vi "CT400_testwrap.vi"() -> ()   [LabVIEW 2013]
uses:
  CT400_Lib/CT400_lib.lvlib
panel:
  out "Error Init":i32
  in  "Laser Type":u32(ring) items=["LS_TunicsPlus", "LS_TunicsPurity", "LS_TunicsReference", "LS_TunicsT100s_HP", "LS_TunicsT100r", "LS_JdsuSws", "LS_Agilent", "NB_SOURCE"]
  out "CT400 Option":string
  out "# Spectral Lines":i32
  out "Spectral lines":dbl[](array[numeric]) format="%#.4f"
  in  "Resolution [pm]":u32=2 max=128 step=1
  out "#Nb of available \ndetectors":i32
  out "# Nb of available\ninputs":i32
  out "# of acquired points":i32
  out "Vext out":dbl format="%.4g"
  out "# of resampled points":i32
  out "Pout-interpolated":dbl[](array[numeric]) format="%.2g"
  out "Detector-interpolated":dbl[](array[numeric]) format="%.2g"
  out "Wavelength re-sampled":dbl[](array[numeric]) format="%.3g"
  in  "Interpolated data":string="Detector1_output-resampled.txt"
  in  "Re-sampled wavelength":string="Wavelength-resampled.txt"
  in  "Detector data":string="Detector1_output.txt"
  in  "Wavelength data":string="Wavelength.txt"
  out "Pout":dbl[](array[numeric]) format="%.2g"
  out "Detector":dbl[](array[numeric]) format="%#.2g"
  out "Wavelength":dbl[](array[numeric]) format="%.4f"
  out "P4 [dBm]":dbl format="%.2g"
  out "P3 [dBm]":dbl format="%.2g"
  out "P2 [dBm]":dbl format="%.2g"
  out "P1 [dBm]":dbl format="%.2g"
  out "Pout [dBm]":dbl format="%.2g"
  out "Error/warning":string
  out "error out":errorcluster
  in  "Start Wavelength [nm]":dbl=1490.0
  in  "Laser power output [mW]":dbl=1.0
  in  "Stop Wavelength [nm]":dbl=1640.0
  in  "Speed [nm/s]":i32=50
  in  "GPIB Address":i32=10
  in  "Upper Wavelength [nm]":dbl=1640.0
  in  "Lower Wavelength [nm]":dbl=1490.0
  in  "error in (no error)":errorcluster
  # "CT400 Settings"
  # "Data files (relative path)"
  # "Laser Settings"
  # "Power on detectors"
  # "Re-sampled Measurements"
  # "Measurements"
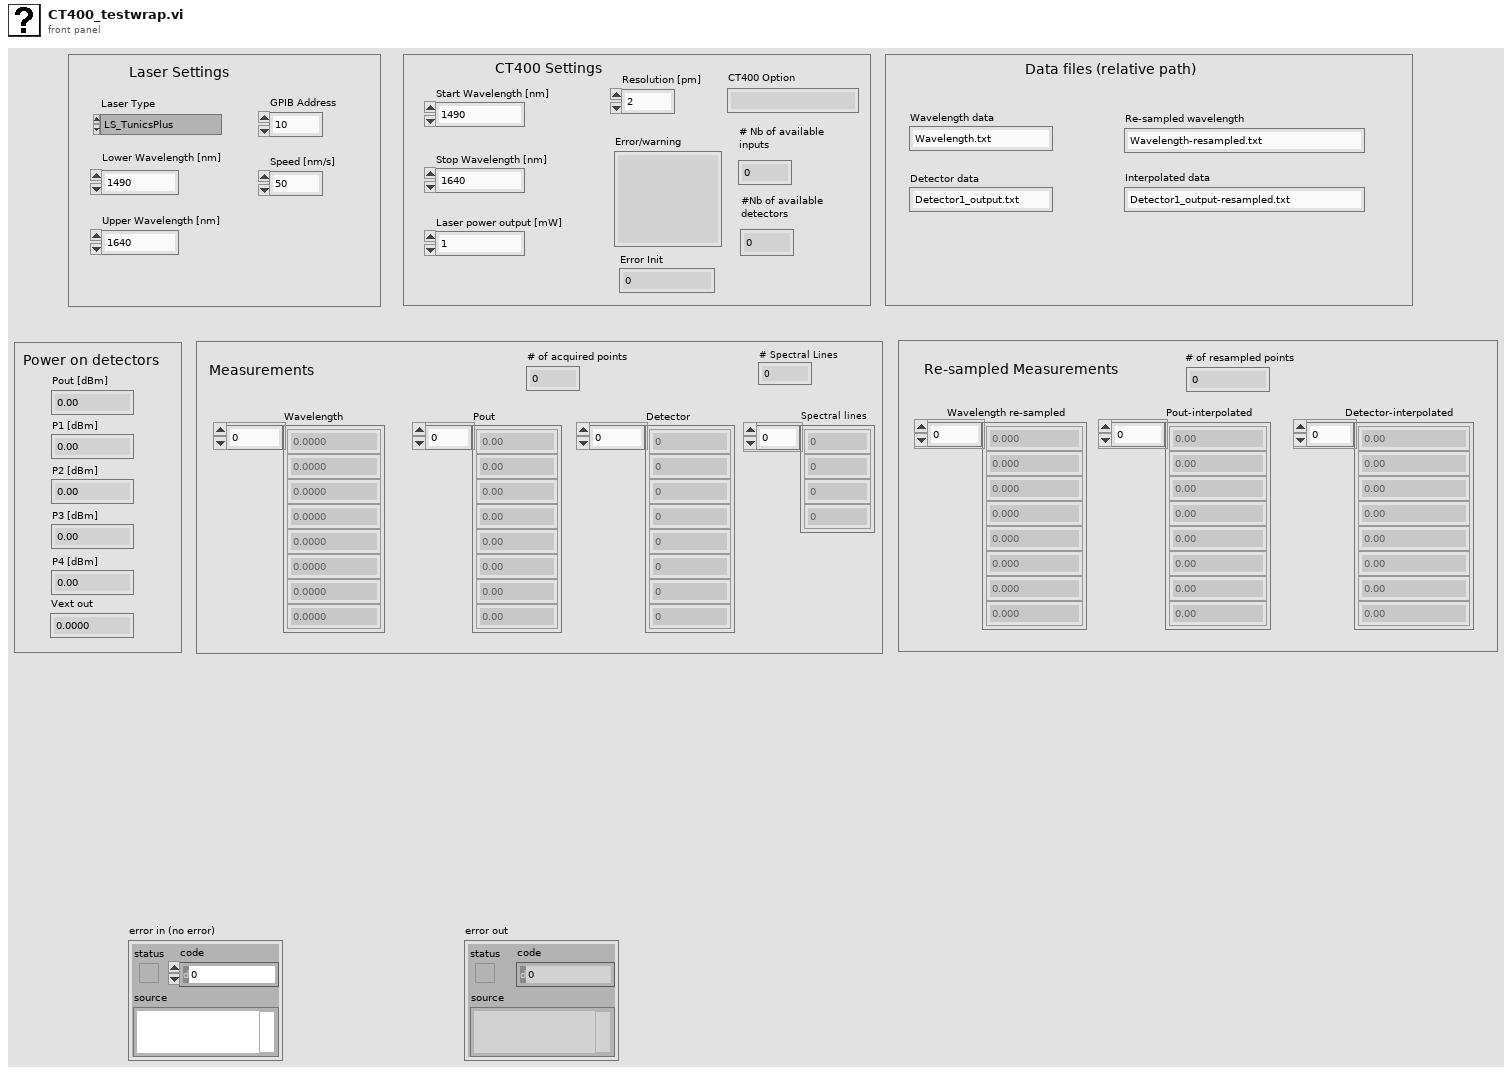
[diagram p1: front panel]
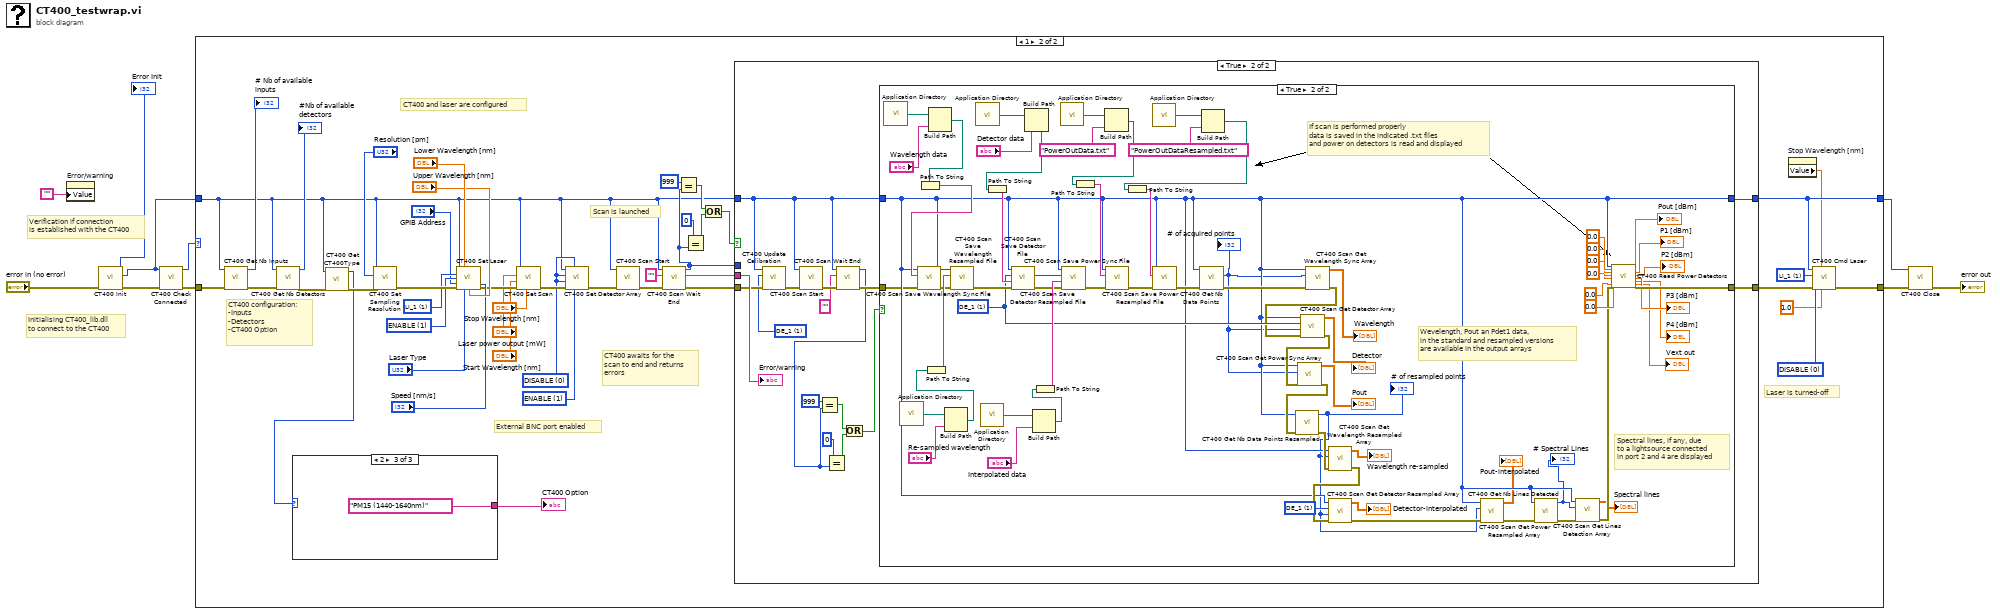
[diagram p0: block diagram]
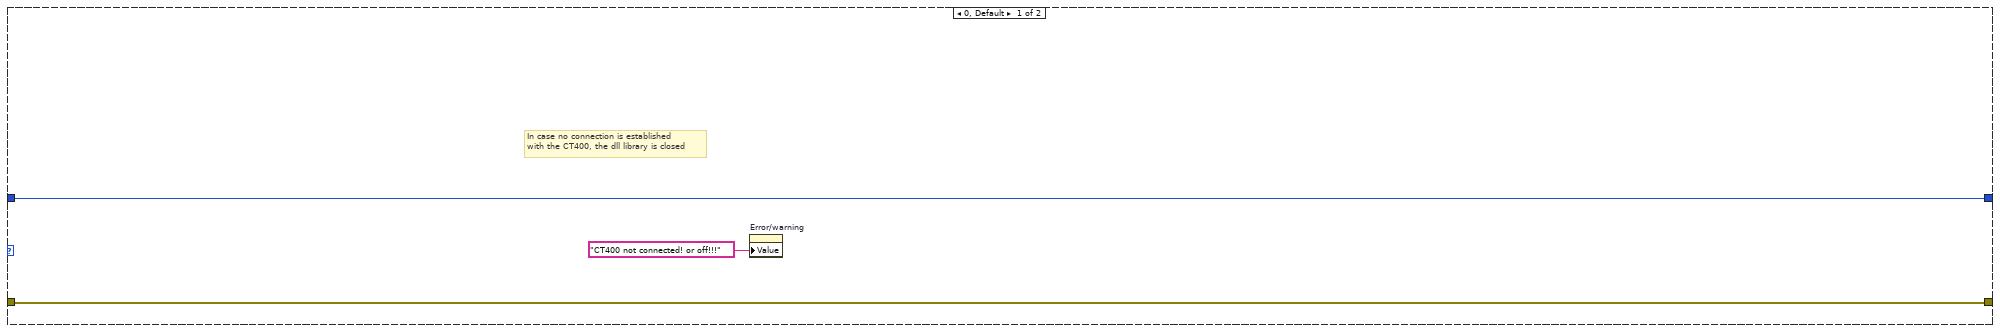
[diagram p2: hidden frame]
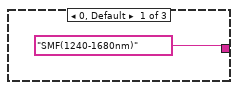
[diagram p3: hidden frame]
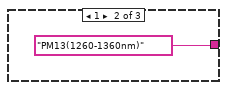
[diagram p4: hidden frame]
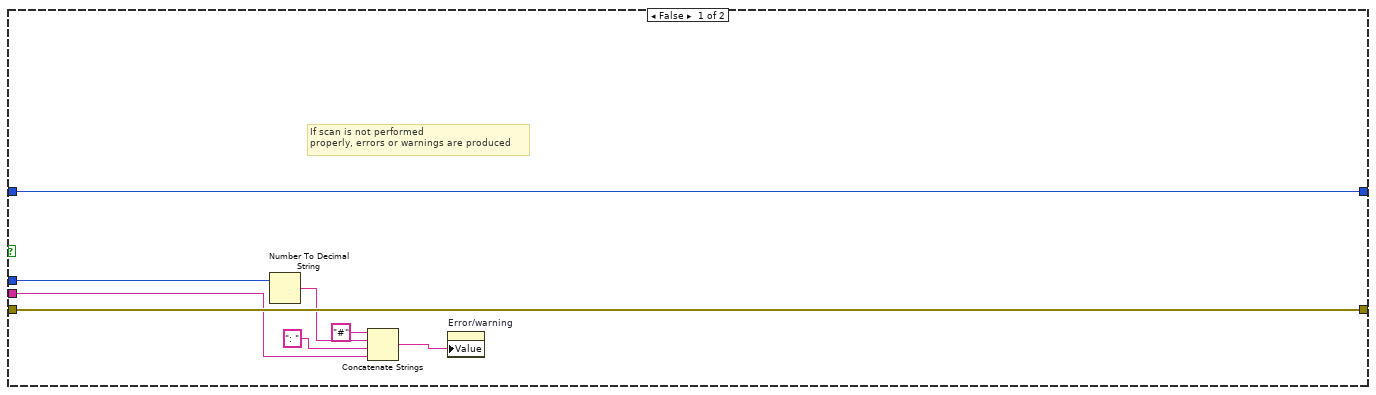
[diagram p5: hidden frame]
diagram:
  # "Verification if connection\nis established with the CT400"
  # "Initialising CT400_lib.dll\nto connect to the CT400"
  n1 = property on="Error/warning" class="Str"("Value"="") -> ()  [unwired: 2 in, 2 out]
  n2 = call "CT400 Init.vi"("error in (no error)"="error in (no error)") -> ("error out"=w9:errorcluster, "function return"=w2:u64, "iError out"=→"Error Init":i32)  [unwired: 8 in]
  n3 = call "CT400 Check Connected.vi"("error in (no error)"=w9, "uiHandle"=w2) -> ("error out"=w7:errorcluster, "function return"=w8:i32)  [unwired: 8 in]
  n4 = case shown="1" w8 {
    tunnel: [w13 w41] -> w6
    tunnel: w7 -> [w13 w25]
    tunnel: [w12 w40] -> w5
    tunnel: w2 -> [w12 w18]
    frame 0, Default {
      # "In case no connection is established\nwith the CT400, the dll library is closed"
      n5 = property on="Error/warning" class="Str"("Value"="CT400 not connected! or off!!!" ("Error/warning")) -> ()  [unwired: 2 in, 2 out]
    }
    frame 1 {
      w14 = u32 1 items=["DISABLE", "ENABLE"] ("eExt")
      w26 = u32 0 items=["DISABLE", "ENABLE"] ("eDect4")
      w38 = u32 1 items=["LI_1"=1, "LI_2"=2, "LI_3"=3, "LI_4"=4] ("eLaser")
      w39 = u32 0 items=["DISABLE", "ENABLE"] ("eEnable")
      w54 = u32 1 items=["DISABLE", "ENABLE"] ("eEnable")
      w55 = u32 1 items=["LI_1"=1, "LI_2"=2, "LI_3"=3, "LI_4"=4] ("eLaser")
      # "CT400 configuration:\n-Inputs\n-Detectors\n-CT400 Option"
      # "External BNC port enabled"
      # "Laser is turned-off"
      # "CT400 awaits for the\nscan to end and returns\nerrors"
      # "Scan is launched"
      # "CT400 and laser are configured"
      n6 = call "CT400 Get Nb Inputs.vi"("error in (no error)"=w25, "uiHandle"=w18) -> ("error out"=w23:errorcluster, "function return"=→"# Nb of available\ninputs":i32)  [unwired: 8 in]
      n7 = call "CT400 Get Nb Detectors.vi"("error in (no error)"=w23, "uiHandle"=w18) -> ("error out"=w19:errorcluster, "function return"=→"#Nb of available \ndetectors":i32)  [unwired: 8 in]
      n8 = call "CT400 Get CT400Type.vi"("error in (no error)"=w19, "uiHandle"=w18) -> ("error out"=w20:errorcluster, "function return"=w17:i32)  [unwired: 8 in]
      n9 = case shown="2" w17 {
        tunnel: ["SMF(1240-1680nm)" ("CT400 Option") "PM13(1260-1360nm)" ("CT400 Option") "PM15 (1440-1640nm)" ("CT400 Option")] -> w16
        frame 0, Default {
        }
        frame 1 {
        }
        frame 2 {
        }
      }
      "CT400 Option" <- w16
      n10 = call "CT400 Set Sampling Resolution.vi"("error in (no error)"=w20, "uiResolution"="Resolution [pm]", "uiHandle"=w18) -> ("error out"=w56:errorcluster)  [unwired: 7 in, 1 out]
      n11 = call "CT400 Set Laser.vi"("uiHandle"=w18, "eLaserType"="Laser Type", "dMaxWavelength"="Upper Wavelength [nm]", "eLaser"=w55, "eEnable"=w54, "iGPIBAdress"="GPIB Address", "error in (no error)"=w56, "dMinWavelength"="Lower Wavelength [nm]", "Speed"="Speed [nm/s]") -> ("error out"=w49:errorcluster)  [unwired: 5 in, 1 out]
      n12 = call "CT400 Set Scan.vi"("dMaxWavelength"="Stop Wavelength [nm]", "error in (no error)"=w49, "dMinWavelength"="Start Wavelength [nm]", "dLaserPower"="Laser power output [mW]", "uiHandle"=w18) -> ("error out"=w28:errorcluster)  [unwired: 5 in, 1 out]
      n13 = call "CT400 Set Detector Array.vi"("eExt"=w14, "eDect4"=w26, "error in (no error)"=w28, "eDect3"=w26, "eDect2"=w26, "uiHandle"=w18) -> ("error out"=w27:errorcluster)  [unwired: 4 in, 1 out]
      n14 = call "CT400 Scan Start.vi"("error in (no error)"=w27, "uiHandle"=w18) -> ("error out"=w29:errorcluster)  [unwired: 8 in, 1 out]
      n15 = call "CT400 Scan Wait End.vi"("error in (no error)"=w29, "tcError"="", "uiHandle"=w18) -> ("error out"=w44:errorcluster, "tcError out"=w43:string, "function return"=w34:i32)  [unwired: 6 in]
      n16 = Equal?(x=999, y=w34) -> (x = y?=w31:bool)
      n17 = Equal?(x=0, y=w34) -> (x = y?=w32:bool)
      n18 = Or(x=w31, y=w32) -> (x .or. y?=w30:bool)
      n19 = case shown="True" w30 {
        tunnel: [w67 w82] -> w42
        tunnel: w18 -> [w66 w77]
        tunnel: w44 -> [w67 w81]
        tunnel: w43 -> [w63 w83]
        tunnel: [w66 w76] -> w40
        tunnel: w34 -> [w65 _]
        frame False {
          # "If scan is not performed \nproperly, errors or warnings are produced"
          n20 = Number To Decimal String(number=w65) -> (decimal integer string=w64:string)  [unwired: 1 in]
          n21 = Concatenate Strings("#" ("string"), w64, ": " ("string"), w63) -> (w62:string)
          n22 = property on="Error/warning" class="Str"("Value"=w62) -> ()  [unwired: 2 in, 2 out]
        }
        frame True {
          w80 = u32 1 items=["DE_1"=1, "DE_2"=2, "DE_3"=3, "DE_4"=4, "DE_5"=5] ("eDetector")
          n23 = call "CT400 Update Calibration.vi"("error in (no error)"=w81, "eDetector"=w80, "uiHandle"=w77) -> ("error out"=w79:errorcluster)  [unwired: 7 in, 1 out]
          n24 = call "CT400 Scan Start.vi"("error in (no error)"=w79, "uiHandle"=w77) -> ("error out"=w78:errorcluster)  [unwired: 8 in, 1 out]
          n25 = call "CT400 Scan Wait End.vi"("error in (no error)"=w78, "tcError"="", "uiHandle"=w77) -> ("error out"=w75:errorcluster, "function return"=w69:i32)  [unwired: 6 in, 1 out]
          n26 = Equal?(x=999, y=w69) -> (x = y?=w73:bool)
          n27 = Equal?(x=0, y=w69) -> (x = y?=w72:bool)
          n28 = Or(x=w73, y=w72) -> (x .or. y?=w68:bool)
          n29 = case shown="True" w68 {
            tunnel: [w84 w150] -> w82
            tunnel: w77 -> [w85 w97]
            tunnel: [w85 w97] -> w76
            tunnel: w75 -> [w84 w96]
            frame False {
            }
            frame True {
              w119 = u32 1 items=["DE_1"=1, "DE_2"=2, "DE_3"=3, "DE_4"=4, "DE_5"=5] ("eDetector")
              w122 = u32 1 items=["DE_1"=1, "DE_2"=2, "DE_3"=3, "DE_4"=4] ("Detector")
              # "Spectral lines, if any, due\nto a lightsource connected\nin port 2 and 4 are displayed"
              # "Wevelength, Pout an Pdet1 data,\nin the standard and resampled versions\nare available in the output arrays"
              # "If scan is performed properly\ndata is saved in the indicated .txt files\nand power on detectors is read and displayed"
              n30 = call <vilib>:"Application Directory.vi"() -> ("Application Directory"=w98:path)
              n31 = call <vilib>:"Application Directory.vi"() -> ("Application Directory"=w133:path)
              n32 = Build Path(base path=w98, name or relative path="Wavelength data") -> (appended path=w137:path)
              n33 = Path To String(path=w137) -> (string=w152:string)
              n34 = call "CT400 Scan Save Wavelength Sync File.vi"("error in (no error)"=w96, "pcPath"=w152, "uiHandle"=w97) -> ("error out"=w129:errorcluster)  [unwired: 6 in, 2 out]
              n35 = Build Path(base path=w133, name or relative path="Re-sampled wavelength") -> (appended path=w131:path)
              n36 = Path To String(path=w131) -> (string=w130:string)
              n37 = call "CT400 Scan Save Wavelength Resampled File.vi"("error in (no error)"=w129, "pcPath"=w130, "uiHandle"=w97) -> ("error out"=w128:errorcluster)  [unwired: 6 in, 2 out]
              n38 = call <vilib>:"Application Directory.vi"() -> ("Application Directory"=w136:path)
              n39 = call <vilib>:"Application Directory.vi"() -> ("Application Directory"=w127:path)
              n40 = Build Path(base path=w136, name or relative path="Detector data") -> (appended path=w134:path)
              n41 = Path To String(path=w134) -> (string=w151:string)
              n42 = call "CT400 Scan Save Detector File.vi"("error in (no error)"=w128, "pcPath"=w151, "eDetector"=w122, "uiHandle"=w97) -> ("error out"=w123:errorcluster)  [unwired: 5 in, 2 out]
              n43 = Build Path(base path=w127, name or relative path="Interpolated data") -> (appended path=w125:path)
              n44 = Path To String(path=w125) -> (string=w124:string)
              n45 = call <vilib>:"Application Directory.vi"() -> ("Application Directory"=w109:path)
              n46 = call "CT400 Scan Save Detector Resampled File.vi"("error in (no error)"=w123, "pcPath"=w124, "eDetector"=w122, "uiHandle"=w97) -> ("error out"=w115:errorcluster)  [unwired: 5 in, 2 out]
              n47 = Build Path(base path=w109, name or relative path="PowerOutData.txt") -> (appended path=w110:path)
              n48 = Path To String(path=w110) -> (string=w106:string)
              n49 = call "CT400 Scan Save Power Sync File.vi"("error in (no error)"=w115, "pcPath"=w106, "uiHandle"=w97) -> ("error out"=w114:errorcluster)  [unwired: 6 in, 2 out]
              n50 = call <vilib>:"Application Directory.vi"() -> ("Application Directory"=w111:path)
              n51 = Build Path(base path=w111, name or relative path="PowerOutDataResampled.txt") -> (appended path=w112:path)
              n52 = Path To String(path=w112) -> (string=w105:string)
              n53 = call "CT400 Scan Save Power Resampled File.vi"("error in (no error)"=w114, "pcPath"=w105, "uiHandle"=w97) -> ("error out"=w113:errorcluster)  [unwired: 6 in, 2 out]
              n54 = call "CT400 Get Nb Data Points.vi"("error in (no error)"=w113, "uiHandle"=w97) -> ("error out"=w117:errorcluster, "iDataPoints out"=w95:i32)  [unwired: 6 in, 2 out]
              "# of acquired points" <- w95
              n55 = call "CT400 Scan Get Wavelength Sync Array.vi"("error in (no error)"=w117, "iArraySize"=w95, "uiHandle"=w97) -> ("error out"=w116:errorcluster, "dArray"=→"Wavelength":dbl[])  [unwired: 6 in, 1 out]
              n56 = call "CT400 Scan Get Detector Array.vi"("error in (no error)"=w116, "iArraySize"=w95, "eDetector"=w122, "uiHandle"=w97) -> ("error out"=w139:errorcluster, "dArray"=→"Detector":dbl[])  [unwired: 5 in, 1 out]
              n57 = call "CT400 Scan Get Power Sync Array.vi"("error in (no error)"=w139, "iArraySize"=w95, "uiHandle"=w97) -> ("error out"=w104:errorcluster, "dArray"=→"Pout":dbl[])  [unwired: 6 in, 1 out]
              n58 = call "CT400 Get Nb Data Points Resampled.vi"("error in (no error)"=w104, "uiHandle"=w97) -> ("error out"=w103:errorcluster, "function return"=w94:i32)  [unwired: 8 in]
              "# of resampled points" <- w94
              n59 = call "CT400 Scan Get Wavelength Resampled Array.vi"("error in (no error)"=w103, "iArraySize"=w94, "uiHandle"=w97) -> ("error out"=w121:errorcluster, "dArray"=→"Wavelength re-sampled":dbl[])  [unwired: 6 in, 1 out]
              n60 = call "CT400 Scan Get Detector Resampled Array.vi"("error in (no error)"=w121, "iArraySize"=w94, "eDetector"=w119, "uiHandle"=w97) -> ("error out"=w120:errorcluster, "dArray"=→"Detector-interpolated":dbl[])  [unwired: 5 in, 1 out]
              n61 = call "CT400 Scan Get Power Resampled Array.vi"("error in (no error)"=w120, "iArraySize"=w94, "uiHandle"=w97) -> ("error out"=w102:errorcluster, "dArray"=→"Pout-interpolated":dbl[])  [unwired: 6 in, 1 out]
              n62 = call "CT400 Get Nb Lines Detected.vi"("error in (no error)"=w102, "uiHandle"=w97) -> ("error out"=w101:errorcluster, "function return"=w87:i32)  [unwired: 8 in]
              "# Spectral Lines" <- w87
              n63 = call "CT400 Scan Get Lines Detection Array.vi"("error in (no error)"=w101, "iArraySize"=w87, "uiHandle"=w97) -> ("error out"=w100:errorcluster, "dArray"=→"Spectral lines":dbl[])  [unwired: 6 in, 1 out]
              n64 = call "CT400 Read Power Detectors.vi"("uiHandle"=w97, "Pout"=0.0, "P1"=0.0, "P2"=0.0, "P3"=0.0, "P4"=0.0, "Vext"=0.0, "error in (no error)"=w100) -> ("Pout out"=→"Pout [dBm]":dbl, "P1 out"=→"P1 [dBm]":dbl, "P2 out"=→"P2 [dBm]":dbl, "P3 out"=→"P3 [dBm]":dbl, "P4 out"=→"P4 [dBm]":dbl, "Vext out"=→"Vext out":dbl, "error out"=w150:errorcluster)  [unwired: 12 in, 1 out]
            }
          }
          "Error/warning" <- w83
        }
      }
      n65 = property on="Stop Wavelength [nm]" class="DigNum (strict)"() -> ("Value"=w36:dbl)  [unwired: 2 in, 2 out]
      n66 = call "CT400 Cmd Laser.vi"("dPower"=1.0, "dWavelength"=w36, "error in (no error)"=w42, "eEnable"=w39, "eLaser"=w38, "uiHandle"=w40) -> ("error out"=w41:errorcluster)  [unwired: 4 in, 1 out]
    }
  }
  n67 = call "CT400 Close.vi"("error in (no error)"=w6, "uiHandle"=w5) -> ("error out"=→"error out":errorcluster)  [unwired: 8 in, 1 out]
